vi "Read File Globals from Calibration Container.vi"(0 "Sequence Ref In":refnum<k7>, 11 "error in":errorcluster) -> (4 "Sequence Ref Out":refnum<k7>, 6 "Variables in Calibration Container":i32, 8 "Calibration Variables":string[](array[string]), 10 "Values":dbl[](array[numeric]), 14 "lookupString":string="DIBCalibration", 15 "error out":errorcluster)   [LabVIEW 2019]
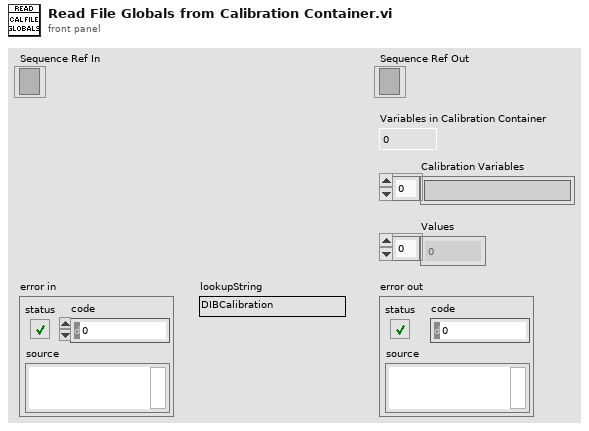
[diagram p1: front panel]
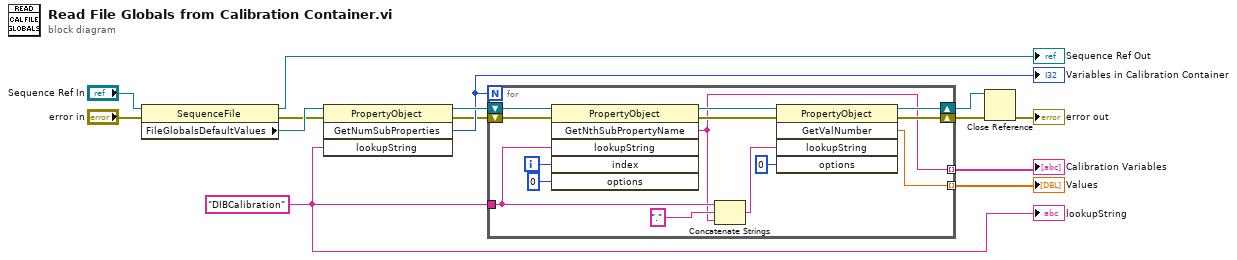
[diagram p0: block diagram]
diagram:
  w12 = "DIBCalibration" ("lookupString")
  n1 = property class="SequenceFile"(reference="Sequence Ref In", error in="error in") -> (reference out=→"Sequence Ref Out":refnum<k7>, error out=w4:errorcluster, "FileGlobalsDefaultValues"=w6:refnum<k7>)
  n2 = invoke class="PropertyObject" method="GetNumSubProperties"(reference=w6, error in=w4, "lookupString"=w12) -> (reference out=w13:refnum<k7>, error out=w7:errorcluster, "GetNumSubProperties"=w10:i32)  [unwired: 1 in, 1 out]
  "Variables in Calibration Container" <- w10
  n3 = for {
    N: w10 -> [_]
    shift-right: [w23] -> w9
    shift-left: w7 -> [w28]
    shift-right: [w21] -> w1
    shift-left: w13 -> [w26]
    tunnel: [w15] -> w11 mode=indexing
    tunnel: w12 -> [w18]
    tunnel: [w20] -> w14 mode=indexing
    i -> [w25]
    n4 = invoke class="PropertyObject" method="GetNthSubPropertyName"(reference=w26, error in=w28, "lookupString"=w18, "index"=w25, "options"=0) -> (reference out=w22:refnum<k7>, error out=w27:errorcluster, "GetNthSubPropertyName"=w15:string)  [unwired: 1 in, 3 out]
    n5 = Concatenate Strings(w18, "." ("string"), w15) -> (w16:string)
    n6 = invoke class="PropertyObject" method="GetValNumber"(reference=w22, error in=w27, "lookupString"=w16, "options"=0) -> (reference out=w21:refnum<k7>, error out=w23:errorcluster, "GetValNumber"=w20:dbl)  [unwired: 1 in, 2 out]
  }
  "Values" <- w14
  "Calibration Variables" <- w11
  n7 = Close Reference(reference=w1, error in (no error)=w9) -> (error out=→"error out":errorcluster)
  "lookupString" <- w12
